vi "8-Byte-to-Byte-Array.vi"(7 "8 Byte in":u64=1091567616 format="%064b") -> (3 "Byte array out":u8[](array[numeric]) format="%08b")   [LabVIEW 2019]
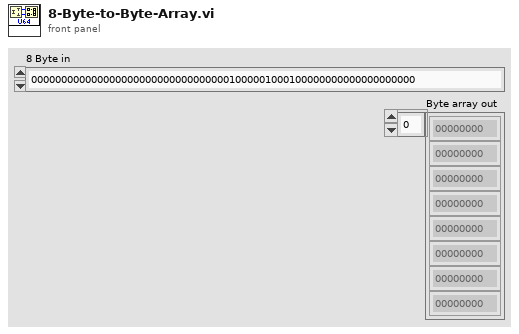
[diagram p1: front panel]
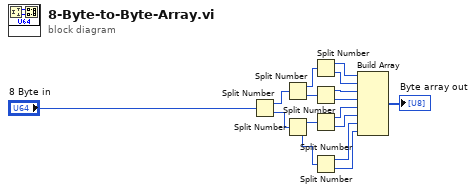
[diagram p0: block diagram]
diagram:
  n1 = Split Number(x="8 Byte in") -> (hi(x)=w13:u32, lo(x)=w14:u32)
  n2 = Split Number(x=w13) -> (hi(x)=w12:u16, lo(x)=w11:u16)
  n3 = Split Number(x=w14) -> (hi(x)=w10:u16, lo(x)=w9:u16)
  n4 = Split Number(x=w12) -> (hi(x)=w8:u8, lo(x)=w7:u8)
  n5 = Split Number(x=w11) -> (hi(x)=w6:u8, lo(x)=w5:u8)
  n6 = Split Number(x=w10) -> (hi(x)=w4:u8, lo(x)=w3:u8)
  n7 = Split Number(x=w9) -> (hi(x)=w2:u8, lo(x)=w1:u8)
  n8 = Build Array(w8, w7, w6, w5, w4, w3, w2, w1) -> (→"Byte array out":u8[])
